vi "start_HB_PollingAgent.vi"() -> ()   [LabVIEW 2009, in "HB_PollingAgent.lvlib"]
uses:
  HB_PollingAgent.lvlib
  HB_PollingAgentVisitor/HB_PollingAgentVisitor.lvclass
  lib.lib/HGF_LVC/HGF_MobileAgentSystem/MoAgSy_AgentBase/MoAgSy_AgentBase.lvclass
  HB_PollingAgent_Factory.lvclass
  lib.lib/HGF_LVC/HGF_BaseClasses/HGF_Factory/HGF_Factory.lvclass
  lib.lib/HGF_LVC/HGF_MobileAgentSystem/MoAgSy_Factory/MoAgSy_Factory.lvclass
  HB_PollingAgent/HB_PollingAgent.lvclass
panel:
  in  "Go":bool
  in  "stop":bool
  out "error out":errorcluster
  in  "journey":string[](array[string])=["psp:\\\\depc210\\depc210_gsi_de0\\Att1", "psp:\\\\denbg029\\denbg029_gsi_de0\\Teacher", "psp:\\\\depc210\\depc210_gsi_de0\\Att1", "psp:\\\\denbg029\\denbg029_gsi_de0\\Teacher", "psp:\\\\depc210\\depc210_gsi_de0\\Att1", "psp:\\\\denbg029\\denbg029_gsi_de0\\Teacher"]
  in  "Question":string="Do you like this LVOOP Course?"
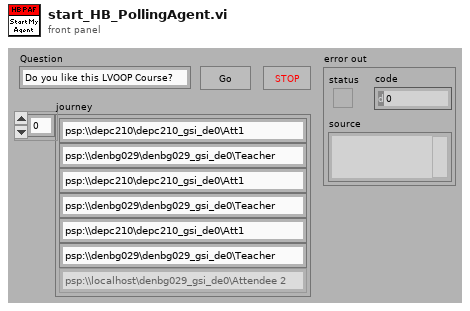
[diagram p1: front panel]
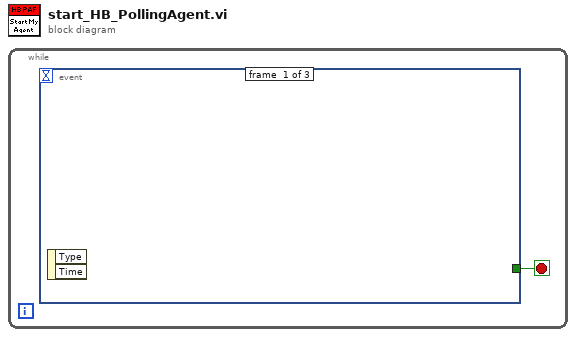
[diagram p0: block diagram]
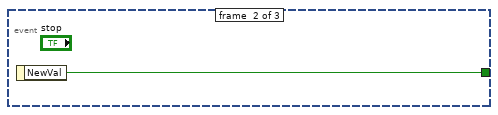
[diagram p2: hidden frame]
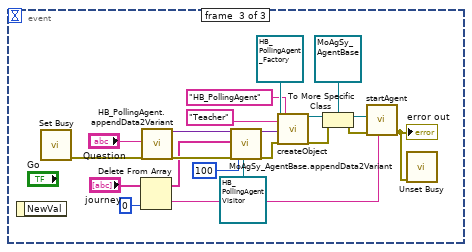
[diagram p3: hidden frame]
diagram:
  n1 = while {
    stop <- w1 stop-if-true
    n2 = event shown="[2] \"Go\": Value Change" {
      selector: _ -> [_ _ _]
      dyn-events: _ -> [_ _ _]
      timeout: _ -> [_ _ _]
      tunnel: [_ w2 _] -> w1
      event #0 {
        n3 = event-data() -> ()  [unwired: 1 in, 2 out]
      }
      event #1 {
        n4 = event-data() -> ("NewVal"=w2:bool)  [unwired: 1 in]
      }
      event #2 {
        n5 = event-data() -> ()  [unwired: 1 in, 1 out]
        n6 = call <vilib>:"Set Busy.vi"() -> ("error out"=w8:errorcluster)  [unwired: 10 in, 1 out]
        n7 = Delete From Array(array="journey", index=0) -> (deleted portion=w4:string, array with subset deleted=w5:string[])  [unwired: 1 in]
        n8 = call "HB_PollingAgent.appendData2Variant.vi"("Question"="Question", "error in (no error)"=w8) -> ("dup initData"=w20:variant, "error out"=w21:errorcluster)  [unwired: 16 in]
        n9 = call "MoAgSy_AgentBase.appendData2Variant.vi"("init"=w20, "journey"=w5, "error in"=w21, "standard Visitor timeout in ms"=100, "standard visitor"=refnum<class "HB_PollingAgentVisitor.lvclass"> refnum ("HB_PollingAgent.lvlib:HB_PollingAgentVisitor.lvclass")) -> ("dup init"=w10:variant, "error out"=w11:errorcluster)  [unwired: 13 in]
        n10 = call "createObject.vi"("HGF_Factory"=refnum<class "HB_PollingAgent_Factory.lvclass"> refnum ("HB_PollingAgent.lvlib:HB_PollingAgent_Factory.lvclass"), "objectName"="Teacher", "initializationData"=w10, "error in (no error)"=w11, "className"="HB_PollingAgent") -> ("HGF_Object"=w12:refnum<class "HGF_Factory.lvclass">, "error out"=w16:errorcluster)  [unwired: 12 in, 1 out]
        n11 = To More Specific Class(target class=refnum<class "MoAgSy_AgentBase.lvclass"> refnum ("MoAgSy_Base.lvlib:MoAgSy_AgentBase.lvclass"), reference=w12, error in=w16) -> (specific class reference=w14:refnum<class "MoAgSy_AgentBase.lvclass">, error out=w15:errorcluster)
        n12 = call "startAgent.vi"("receiver"=w4, "error in (no error)"=w15, "MobileAgent"=w14) -> ("error out"=w7:errorcluster)  [unwired: 8 in]
        "error out" <- w7
        n13 = call <vilib>:"Unset Busy.vi"("error in (no error)"=w7) -> ()  [unwired: 10 in, 1 out]
      }
    }
  }
